vi "Perform Action.vi"(8 "error in":errorcluster, 10 "Input":variant, 11 "DI DAQmx Cont CFG in":refnum<class "DI DAQmx Cont CFG.lvclass">) -> (0 "error out":errorcluster, 2 "Output":variant, 3 "DI DAQmx Cont CFG out":refnum<class "DI DAQmx Cont CFG.lvclass">)   [LabVIEW 2024, in "DI DAQmx Cont CFG.lvclass"]
uses:
  DI DAQmx Cont CFG.lvclass
  DI DAQmx Cont CFG.lvclass/DI DAQmx Cont CFG.ctl
  DAQmx Base CFG/DAQmx Base CFG.lvclass
  Buffers/Buffer Lossless Digital/Buffer Lossless Digital.lvclass
  <vilib>/DAQmx/read.llb/DAQmx Read (Digital 1D Wfm NChan NSamp).vi
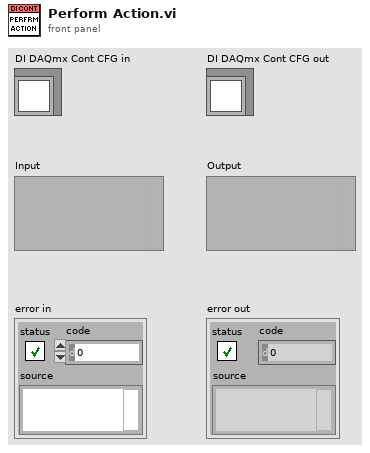
[diagram p1: front panel]
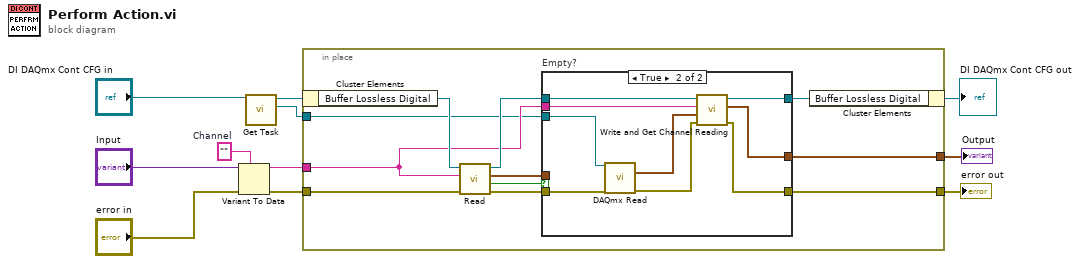
[diagram p0: block diagram]
diagram:
  w10 = ""  # Channel
  n1 = Variant To Data(error in="error in", type=w10, Variant="Input") -> (data=w4:string, error out=w2:errorcluster)
  n2 = call "Get Task.vi"("DAQmx Base CFG in"="DI DAQmx Cont CFG in") -> ("Task"=w1:refnum<k21>, "DAQmx Base CFG out"=w6:refnum<class "DI DAQmx Cont CFG.lvclass">)  [unwired: 9 in]
  n3 = in-place {
    in-place-border: [w22] -> w7
    in-place-border: w4 -> [w16]
    in-place-border: [w19] -> w3
    in-place-border: w2 -> [w17]
    in-place-border: w1 -> [w14]
    n4 = in-place-cluster #1(w6) -> ("Buffer Lossless Digital"=w21:refnum<class "Buffer Lossless Digital.lvclass">)
    n5 = call "Read.vi"("error in"=w17, "Channel"=w16, "Buffer Lossless Bin in"=w21) -> ("error out"=w15:errorcluster, "empty?"=w13:bool, "Digital Waveform"=w12:digitalwaveform, "Buffer Lossless Bin out"=w18:refnum<class "Buffer Lossless Digital.lvclass">)  [unwired: 5 in]
    n6 = case "Empty?" shown="True" w13 {
      tunnel: [w23 w34] -> w22
      tunnel: [w24 w33] -> w20
      tunnel: [w25 w32] -> w19
      tunnel: w18 -> [w24 w31]
      tunnel: w16 -> [_ w30]
      tunnel: w15 -> [w23 w29]
      tunnel: w14 -> [_ w28]
      tunnel: w12 -> [w25 _]
      frame False {
      }
      frame True {
        n7 = call-poly <vilib>:"DAQmx Read.vi"("task/channels in"=w28, "error in"=w29) -> ("data"=w27:digitalwaveform[], "error out"=w26:errorcluster)  [unwired: 11 in, 1 out]
        n8 = call "Write and Get Channel Reading.vi"("error in"=w26, "Readings"=w27, "Channel"=w30, "Buffer Lossless Bin in"=w31) -> ("error out"=w34:errorcluster, "Reading"=w32:digitalwaveform, "Buffer Lossless Bin out"=w33:refnum<class "Buffer Lossless Digital.lvclass">)  [unwired: 5 in]
      }
    }
    n9 = in-place-cluster #1("Buffer Lossless Digital"=w20) -> (→"DI DAQmx Cont CFG out":refnum<class "DI DAQmx Cont CFG.lvclass">)
  }
  "error out" <- w7
  "Output" <- w3
